vi "pid_loop.vi"(0 "Current Pos":dbl, 5 "Desired Pos":dbl, 7 "P":dbl, 9 "I":dbl, 11 "D":dbl, 12 "dt":dbl, 13 "Update PID (F)":bool, 14 "Reset ID":bool) -> (4 "Voltage Output":dbl)   [LabVIEW 2012]
doc: "Standard PID loop. \nSee: http://en.wikipedia.org/wiki/PID_controller"
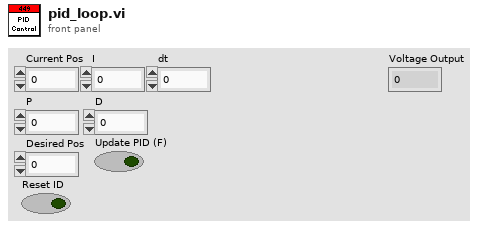
[diagram p1: front panel]
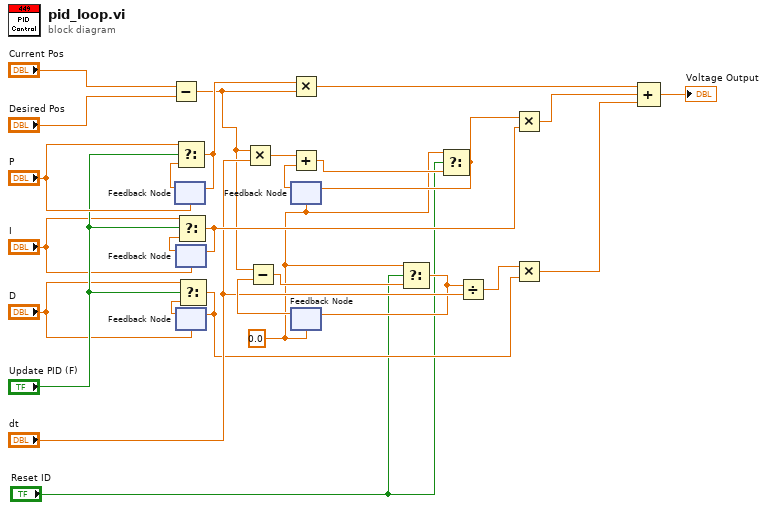
[diagram p0: block diagram]
diagram:
  w2 = 0.0
  n1 = Subtract(x="Current Pos", y="Desired Pos") -> (x-y=w7:dbl)
  n2 = feedback #1("P") -> (w27:dbl)
  n3 = Select(t="P", s="Update PID (F)", f=w27) -> (s? t:f=w18:dbl)
  n4 = feedback-in #1(w18) -> ()
  n5 = feedback #2("I") -> (w24:dbl)
  n6 = feedback #3("D") -> (w25:dbl)
  n7 = Select(t="I", s="Update PID (F)", f=w24) -> (s? t:f=w16:dbl)
  n8 = feedback-in #2(w16) -> ()
  n9 = Select(t="D", s="Update PID (F)", f=w25) -> (s? t:f=w9:dbl)
  n10 = feedback-in #3(w9) -> ()
  n11 = Multiply(x=w7, y="dt") -> (x*y=w14:dbl)
  n12 = Multiply(x=w18, y=w7) -> (x*y=w19:dbl)
  n13 = feedback #4(w2) -> (w17:dbl)
  n14 = Add(x=w14, y=w17) -> (x+y=w6:dbl)
  n15 = feedback #5(w2) -> (w12:dbl)
  n16 = Subtract(x=w7, y=w12) -> (x-y=w4:dbl)
  n17 = Select(t=w2, s="Reset ID", f=w4) -> (s? t:f=w3:dbl)
  n18 = feedback-in #5(w3) -> ()
  n19 = Select(t=w2, s="Reset ID", f=w6) -> (s? t:f=w5:dbl)
  n20 = feedback-in #4(w5) -> ()
  n21 = Divide(x=w3, y="dt") -> (x/y=w10:dbl)
  n22 = Multiply(x=w5, y=w16) -> (x*y=w15:dbl)
  n23 = Multiply(x=w10, y=w9) -> (x*y=w8:dbl)
  n24 = Compound Arithmetic op=ADD(w19, w15, w8) -> (→"Voltage Output":dbl)
